vi "tester.vi"() -> ()   [LabVIEW 2018]
uses:
  build/bin/RCVAnalysis.dll
panel:
  out "FWHM":dbl[](array[numeric])
  out "fullHeight":dbl[](array[numeric])
  out "xValsHalfHeight":dbl[][](array[numeric])
  out "peakArea":dbl[](array[numeric])
  out "xValsFullHeight":dbl[][](array[numeric])
  out "indexes":i32[](array[numeric])
  out "locations":dbl[](array[numeric])
  out "heights":dbl[](array[numeric])
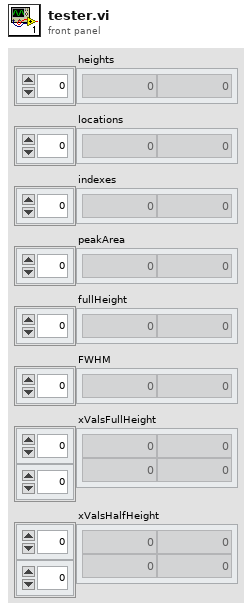
[diagram p1: front panel]
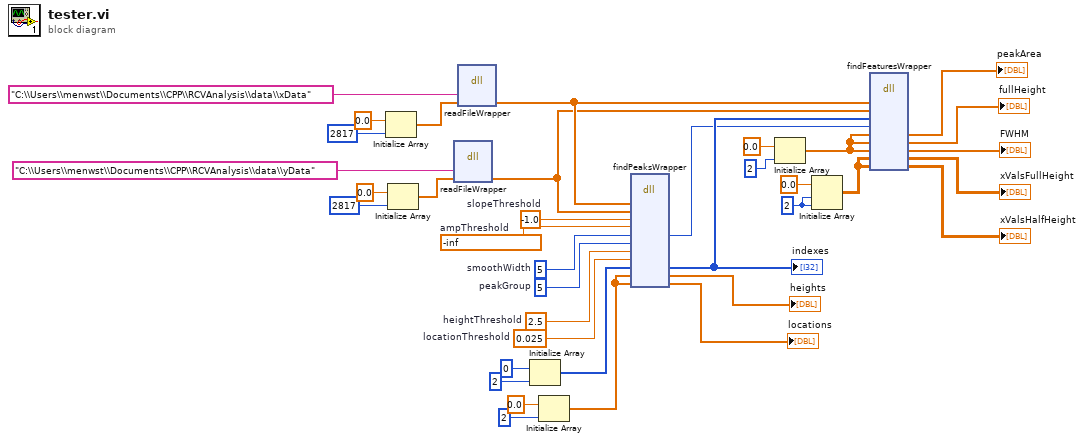
[diagram p0: block diagram]
diagram:
  w17 = 2 ("xnumRows")
  w31 = -inf  # ampThreshold
  w29 = 0.025  # locationThreshold
  w30 = 2.5  # heightThreshold
  w34 = 5  # peakGroup
  w33 = u32 5  # smoothWidth
  w32 = -1.0  # slopeThreshold
  n1 = Initialize Array(0.0 ("element"), 2817 ("dimension size")) -> (w7:dbl[])
  n2 = Initialize Array(0.0 ("element"), 2817 ("dimension size")) -> (w5:dbl[])
  n3 = dll-call lib="C:/Users/menwst/Documents/CPP/RCVAnalysis/build/bin/RCVAnalysis.dll" fn="readFileWrapper"("filename"="C:\\Users\\menwst\\Documents\\CPP\\RCVAnalysis\\data\\yData", "data"=w5) -> ("data"=w1:dbl[])  [unwired: 5 in, 2 out]
  n4 = dll-call lib="C:/Users/menwst/Documents/CPP/RCVAnalysis/build/bin/RCVAnalysis.dll" fn="readFileWrapper"("filename"="C:\\Users\\menwst\\Documents\\CPP\\RCVAnalysis\\data\\xData", "data"=w7) -> ("data"=w6:dbl[])  [unwired: 5 in, 2 out]
  n5 = Initialize Array(0 ("dimension size"), 2 ("dimension size")) -> (w26:i32[])
  n6 = Initialize Array(0.0 ("element"), 2 ("dimension size")) -> (w20:dbl[])
  n7 = dll-call lib="C:/Users/menwst/Documents/CPP/RCVAnalysis/build/bin/RCVAnalysis.dll" fn="findPeaksWrapper"("xdata"=w6, "ydata"=w1, "slopeThreshold"=w32, "ampThreshold"=w31, "smoothWidth"=w33, "peakGroup"=w34, "heightThreshold"=w30, "locationThreshold"=w29, "indexes"=w26, "heights"=w20, "locations"=w20) -> ("smoothWidth"=w21:u32, "indexes"=w22:i32[], "heights"=→"heights":dbl[], "locations"=→"locations":dbl[])  [unwired: 11 in, 2 out]
  "indexes" <- w22
  n8 = Initialize Array(0.0 ("element"), 2 ("xnumRows")) -> (w19:dbl[])
  n9 = Initialize Array(0.0 ("element"), w17, w17) -> (w16:dbl[][])
  n10 = dll-call lib="C:/Users/menwst/Documents/CPP/RCVAnalysis/build/bin/RCVAnalysis.dll" fn="findFeaturesWrapper"("xdata"=w6, "ydata"=w1, "indexes"=w22, "smoothWidth"=w21, "peakArea"=w19, "fullHeight"=w19, "FWHM"=w19, "xValsFullHeight"=w16, "xValsHalfHeight"=w16) -> ("peakArea"=→"peakArea":dbl[], "fullHeight"=→"fullHeight":dbl[], "FWHM"=→"FWHM":dbl[], "xValsFullHeight"=→"xValsFullHeight":dbl[][], "xValsHalfHeight"=→"xValsHalfHeight":dbl[][])  [unwired: 8 in, 2 out]
